vi "Calculate Gyro.vi"(8 "Field Oriented Control?":bool, 11 "Yaw":dbl) -> (3 "Gyro Angle":dbl)   [LabVIEW 2020]
uses:
  Swerve Global Variables.vi
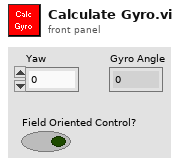
[diagram p1: front panel]
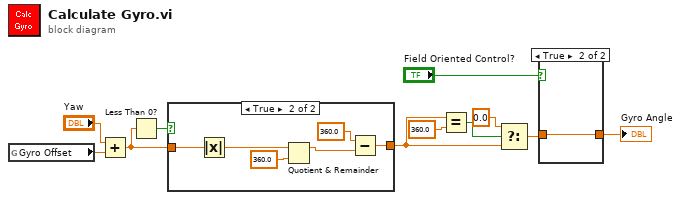
[diagram p0: block diagram]
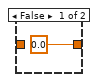
[diagram p2: hidden frame]
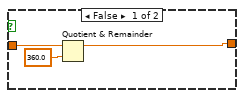
[diagram p3: hidden frame]
diagram:
  n1 = global read "Swerve Global Variables.vi" "Gyro Offset"() -> (w2:dbl)
  n2 = Add(x="Yaw", y=w2) -> (x+y=w1:dbl)
  n3 = Less Than 0?(x=w1) -> (x < 0?=w10:bool)
  n4 = case shown="True" w10 {
    tunnel: w1 -> [w14 w19]
    tunnel: [w12 w16] -> w7
    frame False {
      n5 = Quotient & Remainder(x=w14, y=360.0) -> (x-y*floor(x/y)=w12:dbl)  [unwired: 1 out]
    }
    frame True {
      n6 = Absolute Value(x=w19) -> (abs(x)=w20:dbl)
      n7 = Quotient & Remainder(x=w20, y=360.0) -> (x-y*floor(x/y)=w17:dbl)  [unwired: 1 out]
      n8 = Subtract(x=360.0, y=w17) -> (x-y=w16:dbl)
    }
  }
  n9 = Equal?(x=w7, y=360.0) -> (x = y?=w9:bool)
  n10 = Select(t=0.0, s=w9, f=w7) -> (s? t:f=w6:dbl)
  n11 = case shown="True" "Field Oriented Control?" {
    tunnel: [0.0 w22] -> w4
    tunnel: w6 -> [_ w22]
    frame False {
    }
    frame True {
    }
  }
  "Gyro Angle" <- w4
